vi "get_default_flattened_data.vi"(8 "error in (no error)":errorcluster, 11 "Type Descriptor Enumeration":T1 format="%.0x") -> (0 "error out":errorcluster, 2 "num_bytes":i32, 3 "default_flattened_data":string)   [LabVIEW 2020, in "variant.lvlib" / "variant.lvclass"]
uses:
  variant.lvclass
  Type Descriptor Enumeration.ctl
  variant.lvclass/variant.ctl
  <userlib>/_OpenG.lib/error/error.llb/openg_error.lvlib
  openg_variant.lvlib
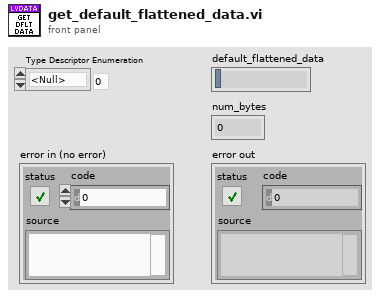
[diagram p1: front panel]
types:
  T1 = typedef "openg_variant.lvlib/Type Descriptor Enumeration.ctl" = enum8{"<Null>", "I8", "I16", "I32", "I64", "U8", "U16", "U32", "U64", "SGL", "DBL", "EXT", "CSG", "CDB", "CXT", "0x0F", "0x10", "0x11", "0x12", "0x13", "0x14", "Enum U8", "Enum U16", "Enum U32", "Enum U64", "SGL PQ", "DBL PQ", "EXT PQ", "CSG PQ", "CDB PQ", "CXT PQ", "0x1F", "0x20", "Boolean", "0x22", "0x23", "0x24", "0x25", "0x26", "0x27", "0x28", "0x29", "0x2A", "0x2B", "0x2C", "0x2D", "0x2E", "0x2F", "String", "0x31", "Path", "Pict", "0x34", "0x35", "0x36", "DAQ", "0x38", "0x39", "0x3A", "0x3B", "0x3C", "0x3D", "0x3E", "0x3F", "Array", "0x41", "0x42", "0x43", "0x44", "0x45", "0x46", "0x47", "0x48", "0x49", "0x4A", "0x4B", "0x4C", "0x4D", "0x4E", "0x4F", "Cluster", "0x51", "0x52", "Variant", "Waveform", "0x55", "0x56", "0x57", "0x58", "0x59", "0x5A", "0x5B", "0x5C", "0x5D", "0x5E", "Fixed Point", "0x60", "0x61", "0x62", "0x63", "0x64", "0x65", "0x66", "0x67", "0x68", "0x69", "0x6A", "0x6B", "0x6C", "0x6D", "0x6E", "0x6F", "Refnum", "0x71", "0x72", "Set Collection", "Map Collection"}
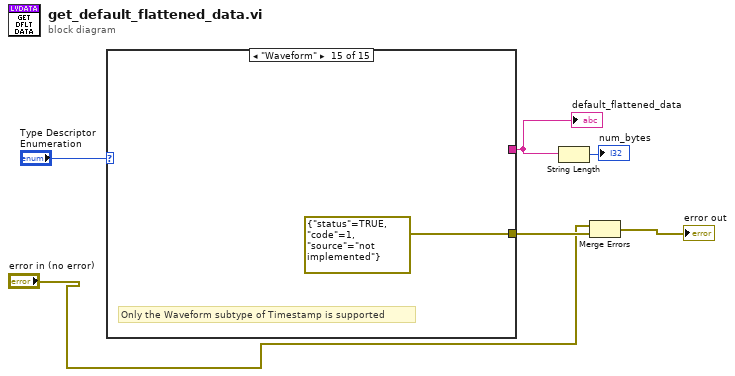
[diagram p0: block diagram]
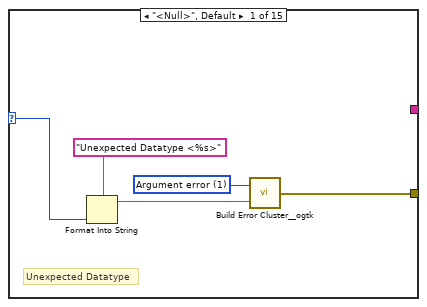
[diagram p2: hidden frame]
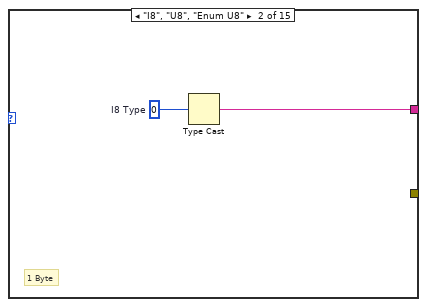
[diagram p3: hidden frame]
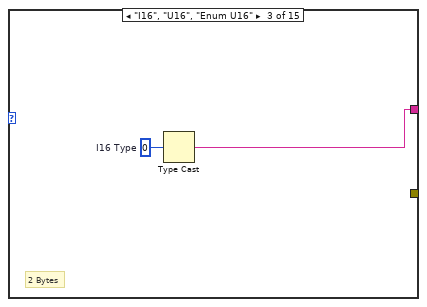
[diagram p4: hidden frame]
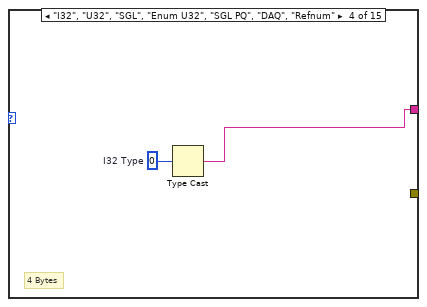
[diagram p5: hidden frame]
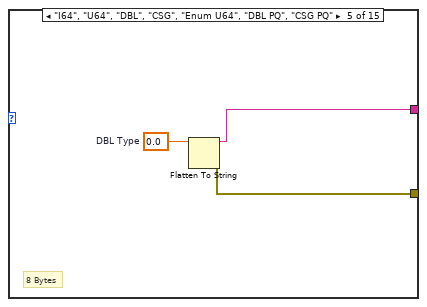
[diagram p6: hidden frame]
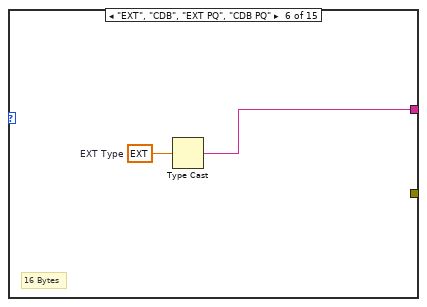
[diagram p7: hidden frame]
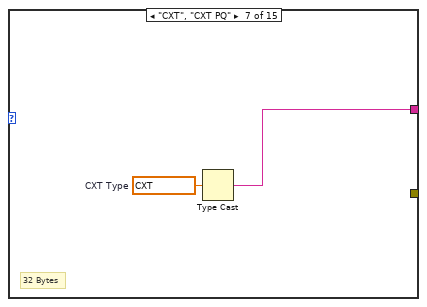
[diagram p8: hidden frame]
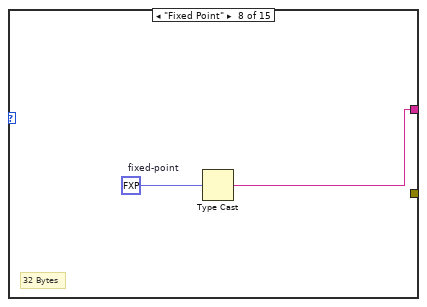
[diagram p9: hidden frame]
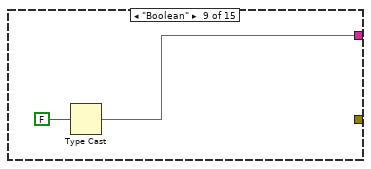
[diagram p10: hidden frame]
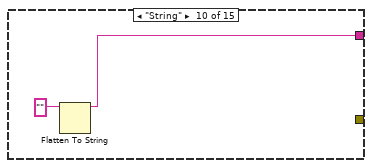
[diagram p11: hidden frame]
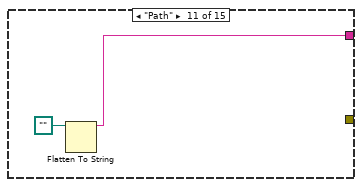
[diagram p12: hidden frame]
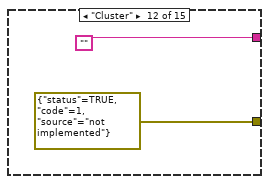
[diagram p13: hidden frame]
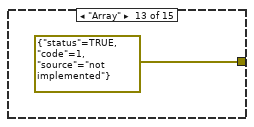
[diagram p14: hidden frame]
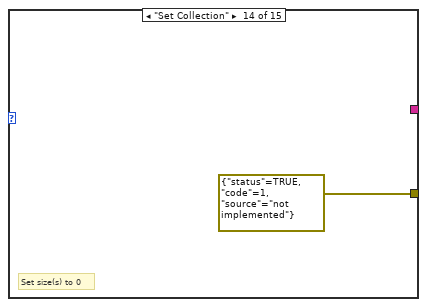
[diagram p15: hidden frame]
diagram:
  n1 = case shown="\"Waveform\"" "Type Descriptor Enumeration" {
    selector: "Type Descriptor Enumeration" -> [w8 _ _ _ _ _ _ _ _ _ _ _ _ _ _]
    tunnel: [w7 _ _ _ w18 _ _ _ _ _ _ errorcluster {"status"=TRUE, "code"=1, "source"="not implemented"} ("error out") errorcluster {"status"=TRUE, "code"=1, "source"="not implemented"} ("error out") errorcluster {"status"=TRUE, "code"=1, "source"="not implemented"} ("error out") errorcluster {"status"=TRUE, "code"=1, "source"="not implemented"} ("error out")] -> w6
    tunnel: [_ w12 w14 w16 w19 w21 w23 w26 w27 w29 w31 "" _ _ _] -> w2
    frame "<Null>", Default {
      w9 = 1 items=["No error", "Argument error", "Memory is full", "Out of zone", "End of file", "File already open", "Generic file I/O error", "File not found", "File permission error", "Disk is full", "Duplicate path", "Too many files open", "System feature not enabled", "Resource file not found", "Cannot add resource", "Resource not found", "Image not found", "Image memory error", "Pen does not exist", "Config type invalid", "Config token not found", "Config parse error", "Config memory error", "Bad external code format", "Bad external code offset", "External code not present", "Null window", "Destroy window error", "Null menu", "Print aborted", "Bad print record", "Print driver error", "Windows error during printing", "Memory error during printing", "Print dialog error", "Generic print error", "Invalid device refnum", "Device not found", "Device parameter error", "Device unit error", "Cannot open device", "Device call aborted", "Generic error", "Cancelled by user", "Object ID too low", "Object ID too high", "Object not in heap", "Unknown heap", "Unknown object (invalid DefProc)", "Unknown object (DefProc not in table)", "Message out of range", "Invalid (null) method", "Unknown message", "Manager call not supported", "Bad address", "Network operation in progress", "Network operation timed out", "Connection is busy", "Network attribute not supported", "Network error", "Address in use", "System out of memory", "Connection aborted", "Connection refused", "Not connected", "Already connected", "Connection closed", "Initialization error (interapplication manager)", "Bad occurrence", "Wait on unbound occurrence handler", "Occurrence queue overflow", "Datalog type conflict", "Unused", "Unrecognized type (interapplication manager)", "Memory corrupt", "Failed to make temporary DLL", "Old CIN version", "Drag socket not found", "Failed to load drop-object", "Failed to register OLE object", "Failed to release OLE object", "Format specifier type mismatch", "Unknown format specifier", "Too few format specifiers", "Too many format specifiers", "Scan failed", "Newer CIN version", "Error converting to variant", "Runtime menu error", "Password tampered", "Variant attribute not found", "Incompatible variant data type", "Event data is not available", "Event Store is not present", "Occurrence is not found", "Event Queue is not created", "Event info is not available", "Refnum passed is NULL", "Error retrieving Class GUID", "Error retrieving CoClass GUID", "Error retrieving TypeLib GUID.", "Bad built application magic bytes.", "Specific driver is different from the specific driver associated with the Logical Name.", "There is no session opened to the class driver.", "Max Error", "MAX - Error with config objects", "MAX - Error loading configuration", "MAX - Group not supported"]
      # "Unexpected Datatype"
      n2 = Format Into String(format string="Unexpected Datatype <%s>" ("Format String"), w8) -> (resulting string=w11:string)  [unwired: 2 in, 1 out]
      n3 = call <userlib>:"Build Error Cluster__ogtk.vi"("String to Prepend to source (\"\")"=w11, "code"=w9) -> ("error out"=w7:errorcluster)
    }
    frame "I8", "U8", "Enum U8" {
      w13 = i8 0  # I8 Type
      # "1 Byte"
      n4 = Type Cast(x=w13) -> (*(type *) &x=w12:string)  [unwired: 1 in]
    }
    frame "I16", "U16", "Enum U16" {
      w15 = i16 0  # I16 Type
      # "2 Bytes"
      n5 = Type Cast(x=w15) -> (*(type *) &x=w14:string)  [unwired: 1 in]
    }
    frame "I32", "U32", "SGL", "Enum U32", "SGL PQ", "DAQ", "Refnum" {
      w17 = 0  # I32 Type
      # "4 Bytes"
      n6 = Type Cast(x=w17) -> (*(type *) &x=w16:string)  [unwired: 1 in]
    }
    frame "I64", "U64", "DBL", "CSG", "Enum U64", "DBL PQ", "CSG PQ" {
      w20 = 0.0  # DBL Type
      # "8 Bytes"
      n7 = Flatten To String(anything=w20) -> (data string=w19:string, error out=w18:errorcluster)  [unwired: 3 in, 1 out]
    }
    frame "EXT", "CDB", "EXT PQ", "CDB PQ" {
      w22 = ext 0.0  # EXT Type
      # "16 Bytes"
      n8 = Type Cast(x=w22) -> (*(type *) &x=w21:string)  [unwired: 1 in]
    }
    frame "CXT", "CXT PQ" {
      w24 = cxt 0.0+0.0i  # CXT Type
      # "32 Bytes"
      n9 = Type Cast(x=w24) -> (*(type *) &x=w23:string)  [unwired: 1 in]
    }
    frame "Fixed Point" {
      w25 = fxp<+/-,32,16> 0.0  # fixed-point
      # "32 Bytes"
      n10 = Type Cast(x=w25) -> (*(type *) &x=w26:string)  [unwired: 1 in]
    }
    frame "Boolean" {
      n11 = Type Cast(x=FALSE ("status")) -> (*(type *) &x=w27:string)  [unwired: 1 in]
    }
    frame "String" {
      n12 = Flatten To String(anything="") -> (data string=w29:string)  [unwired: 3 in, 2 out]
    }
    frame "Path" {
      n13 = Flatten To String(anything=path "") -> (data string=w31:string)  [unwired: 3 in, 2 out]
    }
    frame "Cluster" {
    }
    frame "Array" {
    }
    frame "Set Collection" {
      # "Set size(s) to 0"
    }
    frame "Waveform" {
      # "Only the Waveform subtype of Timestamp is supported"
    }
  }
  "default_flattened_data" <- w2
  n14 = String Length(string=w2) -> (length=→"num_bytes":i32)
  n15 = Merge Errors("error in (no error)", w6) -> (→"error out":errorcluster)
